vi "PRIME Insert FITS header before image.vi"() -> ()   [LabVIEW 2020, in "PRIME Detector.lvclass"]
uses:
  PRIME Detector.lvclass
  Detector Image typedef cluster.ctl
  Detector Class.lvclass
  RIMAS Detector Server Config.ctl
  RIMAS Observation Config.ctl
  Detector enum Detector Integration Mode.ctl
  RIMAS Detector Config.ctl
panel:
  in  "FITS Detector Settings":T1
  in  "Detector Config":T2={"Detector"=0, "Offsets"=[[0, 0, 0, 0, 0, 0, 0, 0, 0, 0, 0, 0, 0, 0, 0, 0, 0, 0, 0, 0, 0, 0, 0, 0, 0, 0, 0, 0, 0, 0, 0, 0]], "Detector Computer"={"Machine"="192.168.121.11", "Password"="rSL!nux23456", "FITS File Path"="", "Port"=44444, "Header Path"="", "Name"=""}, "FITS hdr template0"=path "", "FITS hdr template1"=path "", "FITS Data File Path"=path "", "FITS Detector Settings"={"Exp Time Short"=0.0, "# of Frames"=0.0, "Exp Time Long"=0.0, "# of Groups"=0.0, "Object Name"="", "Object"="", "Obs Type"="", "Image Type"="", "Observer"="", "Observer Affiliation"=""}, "Sim Folder"=path "", "Integration Mode"=enum."SSR", "Integration Time"=0.0, "Frame Int Time"=0.0} {"Offsets" format="%04x"; "Detector" items=["0", "1", "2"]}
  out "Images out":T5[](array[typedef]) {"Detector #" items=["None", "YJ", "HK"]}
  in  "Images":T5[](array[typedef]) {"Detector #" items=["None", "YJ", "HK"]}
  # "sec"
  # "sec"
  # "sec"
  # "sec"
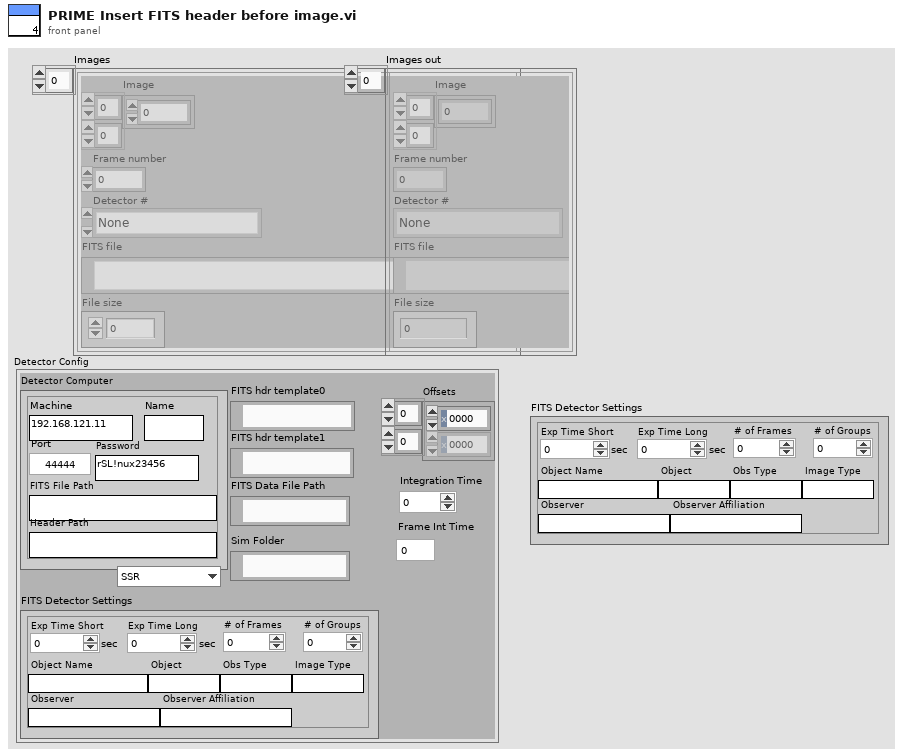
[diagram p1: front panel]
types:
  T1 = typedef "RIMAS Observation Config.ctl" = cluster{"Exp Time Short":dbl, "# of Frames":dbl, "Exp Time Long":dbl, "# of Groups":dbl, "Object Name":string, "Object":string, "Obs Type":string, "Image Type":string, "Observer":string, "Observer Affiliation":string}
  T2 = typedef "RIMAS Detector Config.ctl" = cluster{"Detector":u16, "Offsets":u16[][], "Detector Computer":T3, "FITS hdr template0":path, "FITS hdr template1":path, "FITS Data File Path":path, "FITS Detector Settings":T1, "Sim Folder":path, "Integration Mode":T4, "Integration Time":dbl, "Frame Int Time":dbl}
  T3 = typedef "RIMAS Detector Server Config.ctl" = cluster{"Machine":string, "Password":string, "FITS File Path":string, "Port":u16, "Header Path":string, "Name":string}
  T4 = typedef "Detector enum Detector Integration Mode.ctl" = enum16{"SSR", "CDS", "MEAN", "MEDIAN", "MODE", "MIIN", "MAX"}
  T5 = typedef "Detector Class.lvclass/Detector Image typedef cluster.ctl" = cluster{"Image":sgl[][], "Frame number":i32, "Detector #":u16, "FITS file":path, "File size":i64}
  T6 = typedef "gfitsio.lvlib/gfitsio-refnum.ctl" = refnum<k1>
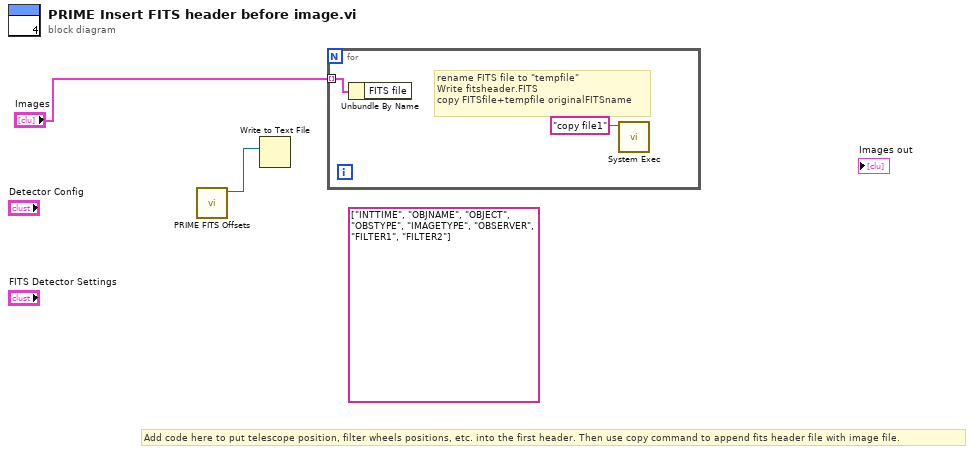
[diagram p0: block diagram]
diagram:
  (unwired) string[] ["INTTIME", "OBJNAME", "OBJECT", "OBSTYPE", "IMAGETYPE", "OBSERVER", "FILTER1", "FILTER2"]
  # "Add code here to put telescope position, filter wheels positions, etc. into the first header. Then use copy command to append fits header file with image file."
  n1 = call "PRIME FITS Offsets.vi"() -> ("gfits refnum out"=w1:T6)  [unwired: 10 in, 1 out]
  n2 = Write to Text File(text=w1) -> ()  [unwired: 3 in, 3 out]
  n3 = for {
    tunnel: "Images" -> [w4] mode=indexing
    # "rename FITS file to \"tempfile\"\nWrite fitsheader.FITS \ncopy FITSfile+tempfile originalFITSname"
    n4 = Unbundle By Name(w4) -> ()  [unwired: 1 out]
    n5 = call <vilib>:"System Exec.vi"("command line"="copy file1") -> ()  [unwired: 7 in, 4 out]
  }
